vi "DrawRectangleOnImageGreyscale.vi"(4 "Thickness (Default: 1)":i32=1, 6 "Colour":u8=255, 7 "OpenCV Line Type (Default LINE_8)":T2=enum."LINE_8", 8 "error in (no error)":errorcluster, 9 "Point B":T1, 10 "Point A":T1, 11 "Greyscale Image":refnum<data-value>) -> (0 "error out":errorcluster, 3 "Greyscale Image (Duplicate)":refnum<data-value>)   [LabVIEW 2020, in "g_ar_toolkit.image.lvlib"]
uses:
  g_ar_toolkit.image.lvlib
  7e6fb015-3761-4366-a0a7-e436eb229083.vi
  Line Type.ctl
  Image Point (Fixed).ctl
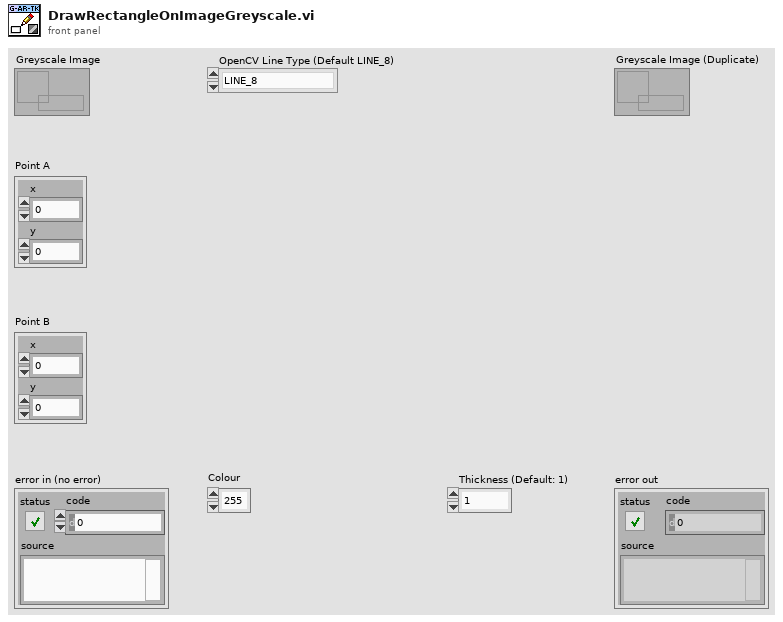
[diagram p1: front panel]
types:
  T1 = typedef "g_ar_toolkit.image.lvlib/Image Point (Fixed).ctl" = cluster{"x":i32, "y":i32}
  T2 = typedef "g_ar_toolkit.image.lvlib/Line Type.ctl" = enum8{"FILLED", "LINE_4", "LINE_8", "LINE_AA"}
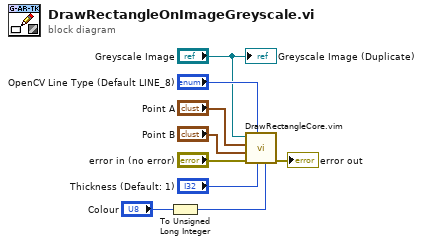
[diagram p0: block diagram]
diagram:
  n1 = To Unsigned Long Integer(number="Colour") -> (unsigned 32bit integer=w2:u32)
  n2 = call "DrawRectangleCore.vim"("Colour"=w2, "Thickness"="Thickness (Default: 1)", "OpenCV Line Type"="OpenCV Line Type (Default LINE_8)", "error in (no error)"="error in (no error)", "Point B"="Point B", "Point A"="Point A", "Src"="Greyscale Image") -> ("error out"=→"error out":errorcluster)  [unwired: 4 in]
  "Greyscale Image (Duplicate)" <- "Greyscale Image"
